vi "Low Level SubVI.vi"(8 "error in (no error)":errorcluster, 10 "write buffer":string, 11 "VISA Refnum in":refnum<visa-resource-name>) -> (0 "error out":errorcluster, 2 "output 1":u16, 3 "VISA Refnum out":refnum<visa-resource-name>)   [LabVIEW 2015]
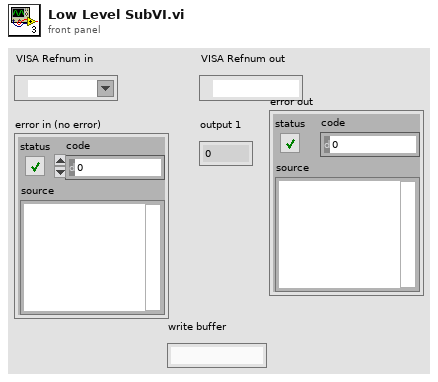
[diagram p1: front panel]
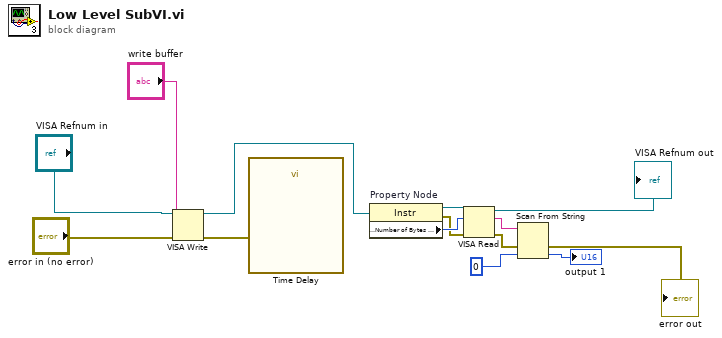
[diagram p0: block diagram]
diagram:
  n1 = VISA Write(VISA resource name="VISA Refnum in", write buffer="write buffer", error in (no error)="error in (no error)") -> (VISA resource name out=w6:refnum<visa-resource-name>, error out=w5:errorcluster)  [unwired: 1 out]
  n2 = call "Time Delay"("error in (no error)"=w5) -> ()  [unwired: 10 in, 1 out]
  n3 = property on="Property Node" class="Instr"(reference=w6) -> (reference out=w9:refnum<visa-resource-name>, error out=w7:errorcluster, "Serial Settings:Number of Bytes at Serial Port"=w8:u32)  [unwired: 1 in]
  n4 = VISA Read(VISA resource name=w9, byte count=w8, error in (no error)=w7) -> (VISA resource name out=→"VISA Refnum out":refnum<visa-resource-name>, read buffer=w11:string, error out=w10:errorcluster)  [unwired: 1 out]
  n5 = Scan From String "Scan From String"(input string=w11, error in=w10, default 1=u16 0 ("default value 1")) -> (error out=→"error out":errorcluster, output 1=→"output 1":u16)  [unwired: 2 in, 2 out]
